vi "frw_get_extra_param.vi"(11 "Path":path) -> (2 "extra_string":string, 3 "channels_str":string)   [LabVIEW 2013]
doc: "Reads parameters form EEG file, CSV or EDF"
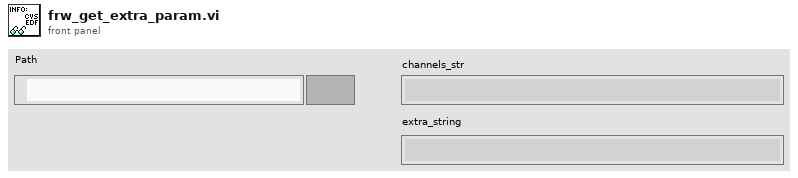
[diagram p1: front panel]
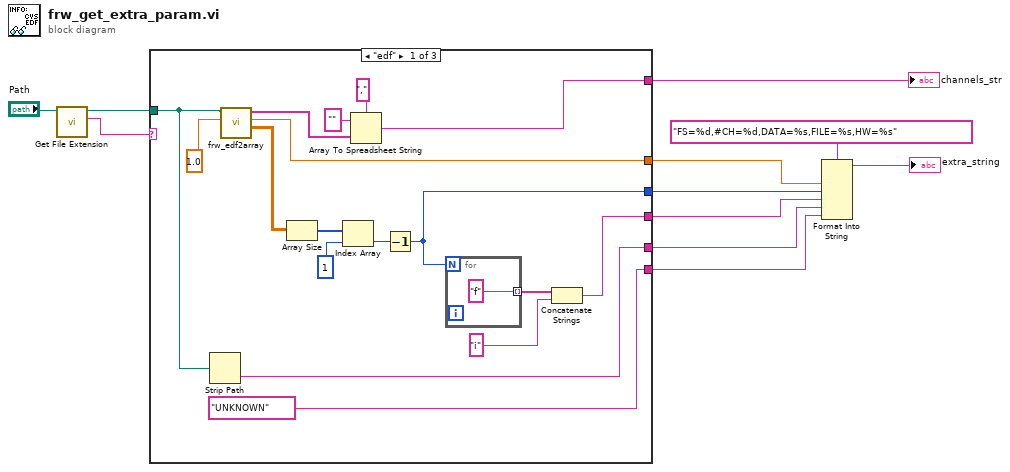
[diagram p0: block diagram]
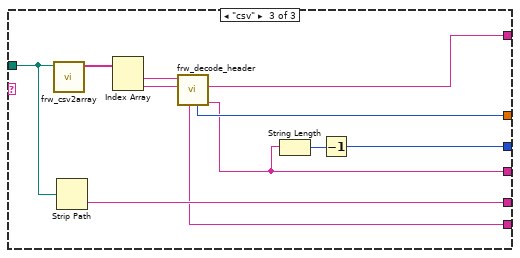
[diagram p3: hidden frame]
diagram:
  n1 = call <vilib>:"Get File Extension.vi"("file"="Path") -> ("lowercase file extension"=w10:string, "dup file"=w9:path)  [unwired: 7 in, 2 out]
  n2 = case shown="\"edf\"" w10 {
    tunnel: w9 -> [w14 _ w32]
    tunnel: [w26 _ w37] -> w8
    tunnel: [w23 _ w36] -> w6
    tunnel: [w15 _ w35] -> w5
    tunnel: [w18 _ w33] -> w4
    tunnel: [w13 _ w31] -> w2
    tunnel: ["UNKNOWN" _ w30] -> w1
    frame "edf" {
      n3 = Strip Path(path=w14) -> (name=w13:string)  [unwired: 1 out]
      n4 = call "frw_edf2array.vi"("block size (3600s)"=1.0 ("block size"), "file path"=w14) -> ("2D array"=w22:dbl[][], "fs"=w23:dbl, "channel names out"=w24:string[])  [unwired: 7 in]
      n5 = Array Size(array=w22) -> (size(s)=w21:i32[])
      n6 = Index Array(array=w21, index=1) -> (element=w19:i32)
      n7 = Array To Spreadsheet String(delimiter (Tab)=",", array=w24, 3:"" ("format string")) -> (spreadsheet string=w26:string)
      n8 = Decrement(x=w19) -> (x-1=w18:i32)
      n9 = for {
        N: w18 -> [_]
        tunnel: ["f"] -> w17 mode=indexing
      }
      n10 = Concatenate Strings(w17, "i") -> (w15:string)
    }
    frame Default {
    }
    frame "csv" {
      n11 = call "frw_csv2array.vi"("file path"=w32) -> ("headerarray"=w40:string[])  [unwired: 7 in, 3 out]
      n12 = Strip Path(path=w32) -> (name=w31:string)  [unwired: 1 out]
      n13 = Index Array(array=w40) -> (element #1=w39:string, element #2=w38:string)  [unwired: 2 in]
      n14 = call "frw_decode_header.vi"("header2"=w38, "header1"=w39) -> ("tags"=w35:string, "chLabels"=w37:string, "fs"=w36:i32, "hardware"=w30:string)  [unwired: 4 in, 2 out]
      n15 = String Length(string=w35) -> (length=w34:i32)
      n16 = Decrement(x=w34) -> (x-1=w33:i32)
    }
  }
  "channels_str" <- w8
  n17 = Format Into String(format string="FS=%d,#CH=%d,DATA=%s,FILE=%s,HW=%s", w6, w4, w5, w2, w1) -> (resulting string=→"extra_string":string)  [unwired: 2 in, 1 out]
